vi "Registry - register at runtime.vi"(8 "error in (no error)":errorcluster) -> (0 "error out":errorcluster)   [LabVIEW 2026, in "Tests.lvlib"]
doc: "Verifies that unregistering one appender stops its delivery while the others keep receiving. Registers three queue-mode relay appenders, logs once (all three receive), unregisters relayB, logs again, and asserts the two survivors receive the second message and relayB receives nothing. Exercises the IDAbsent barrier in UnregisterAppender.\n\nImplements LMBR-T-032 -> SRS-020. Assert-level IDs: Test-ID-Assert-Checklist.md."
uses:
  Tests.lvlib
  src/TypeDefs/Severity.ctl
  <vilib>/addons/_JKI Toolkits/Caraya/classes/Assert/Assert Equal Value_Variant.vi
  <vilib>/addons/_JKI Toolkits/Caraya/classes/Assert/Assert True.vi
  <vilib>/addons/_JKI Toolkits/Caraya/classes/Test/Test.lvclass
  src/Lumberjack.lvlib
  src/Public/Logger.lvclass/Logger.lvclass
  <vilib>/addons/_JKI Toolkits/Caraya/classes/Assert/Assert.lvclass
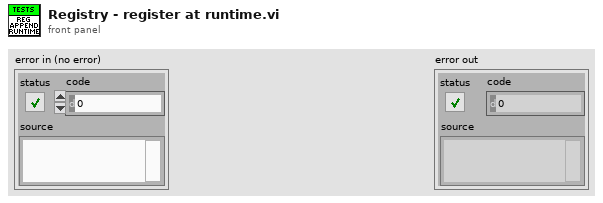
[diagram p1: front panel]
types:
  T1 = typedef "Lumberjack.lvlib/Severity.ctl" = enum16{"OFF", "FATAL", "ERROR", "WARN", "INFO", "DEBUG", "TRACE", "ALL"}
  T2 = typedef "Lumberjack.lvlib/Statement.ctl" = cluster{"timestamp":timestamp, "level":T1, "sourceTag":string, "originVI":string, "message":string}
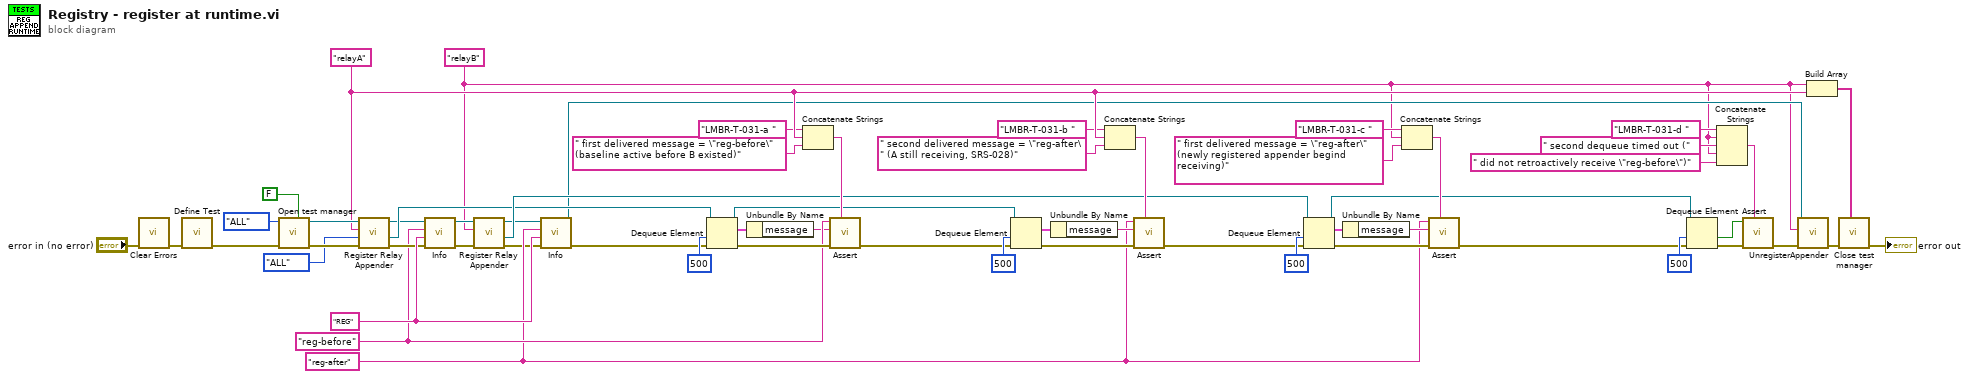
[diagram p0: block diagram]
diagram:
  w13 = "reg-after" ("message")
  w8 = "relayB"
  w38 = "relayA"
  w40 = "REG" ("sourceTag")
  w25 = "reg-before" ("message")
  n1 = call <vilib>:"Clear Errors.vi"("error in (no error)"="error in (no error)") -> ("error out"=w1:errorcluster)  [unwired: 5 in, 1 out]
  n2 = call <vilib>:"Define Test.vi"("error in (no error)"=w1) -> ("error out"=w60:errorcluster)  [unwired: 9 in, 1 out]
  n3 = call "Open test manager.vi"("enableDefaultFile"=FALSE, "error in (no error)"=w60, "globalThreshold"=Severity."ALL") -> ("error out"=w57:errorcluster, "Logger out"=w58:refnum<class "Logger.lvclass">)  [unwired: 7 in]
  n4 = call "Register Relay Appender.vi"("error in (no error)"=w57, "threshold"=Severity."ALL", "id in"=w38, "Logger in"=w58) -> ("error out"=w30:errorcluster, "relayQueue"=w37:refnum<queue>, "Logger out"=w29:refnum<class "Logger.lvclass">)  [unwired: 4 in, 1 out]
  n5 = call "Info.vi"("error in (no error)"=w30, "sourceTag"=w40, "message"=w25, "Logger in"=w29) -> ("error out"=w5:errorcluster, "Logger out"=w28:refnum<class "Logger.lvclass">)  [unwired: 6 in]
  n6 = call "Register Relay Appender.vi"("error in (no error)"=w5, "id in"=w8, "Logger in"=w28) -> ("error out"=w4:errorcluster, "relayQueue"=w39:refnum<queue>, "Logger out"=w27:refnum<class "Logger.lvclass">)  [unwired: 5 in, 1 out]
  n7 = call "Info.vi"("error in (no error)"=w4, "sourceTag"=w40, "message"=w13, "Logger in"=w27) -> ("error out"=w3:errorcluster, "Logger out"=w26:refnum<class "Logger.lvclass">)  [unwired: 6 in]
  n8 = Dequeue Element(queue=w37, timeout in ms (-1)=500, error in (no error)=w3) -> (queue out=w20:refnum<queue>, element=w52:T2, error out=w53:errorcluster)  [unwired: 1 out]
  n9 = Unbundle By Name(w52) -> ("message"=w24:string)
  n10 = Concatenate Strings("LMBR-T-031-a " ("string"), w38, " first delivered message = \"reg-before\" (baseline active before B existed)" ("Label")) -> (w55:string)
  n11 = call-poly <vilib>:"Assert.vi"("Label"=w55, "error in (no error)"=w53, "Actual"=w24, "Expected"=w25) -> ("error out"=w22:errorcluster)  [unwired: 6 in, 1 out]
  n12 = Dequeue Element(queue=w20, timeout in ms (-1)=500, error in (no error)=w22) -> (element=w16:T2, error out=w21:errorcluster)  [unwired: 2 out]
  n13 = Unbundle By Name(w16) -> ("message"=w15:string)
  n14 = Concatenate Strings("LMBR-T-031-b " ("string"), w38, " second delivered message = \"reg-after\" (A still receiving, SRS-028)" ("Label")) -> (w54:string)
  n15 = call-poly <vilib>:"Assert.vi"("Label"=w54, "error in (no error)"=w21, "Actual"=w15, "Expected"=w13) -> ("error out"=w48:errorcluster)  [unwired: 6 in, 1 out]
  n16 = Dequeue Element(queue=w39, timeout in ms (-1)=500, error in (no error)=w48) -> (queue out=w9:refnum<queue>, element=w49:T2, error out=w14:errorcluster)  [unwired: 1 out]
  n17 = Unbundle By Name(w49) -> ("message"=w50:string)
  n18 = Concatenate Strings("LMBR-T-031-c " ("string"), w8, " first delivered message = \"reg-after\" (newly registered appender begind receiving)" ("Label")) -> (w10:string)
  n19 = call-poly <vilib>:"Assert.vi"("Label"=w10, "error in (no error)"=w14, "Actual"=w50, "Expected"=w13) -> ("error out"=w42:errorcluster)  [unwired: 6 in, 1 out]
  n20 = Dequeue Element(queue=w9, timeout in ms (-1)=500, error in (no error)=w42) -> (timed out?=w44:bool, error out=w45:errorcluster)  [unwired: 2 out]
  n21 = Concatenate Strings("LMBR-T-031-d " ("string"), w8, " second dequeue timed out (" ("Label"), w8, " did not retroactively receive \"reg-before\")" ("string")) -> (w46:string)
  n22 = call-poly <vilib>:"Assert.vi"("Label"=w46, "error in (no error)"=w45, "True?"=w44) -> ("error out"=w6:errorcluster)  [unwired: 7 in, 1 out]
  n23 = call "UnregisterAppender.vi"("error in (no error)"=w6, "id"=w8, "Logger in"=w26) -> ("error out"=w17:errorcluster)  [unwired: 7 in, 1 out]
  n24 = Build Array(w8, w38) -> (w36:string[])
  n25 = call "Close test manager.vi"("queueIDList"=w36, "error in (no error)"=w17) -> ("error out"=→"error out":errorcluster)  [unwired: 7 in]
